vi "Get Brewer Palette Colors by Name (#Colors).vi"(11 "Brewer Palette Name (# Colors)":string) -> (0 "Found?":bool, 3 "Color Array":u32[](array[numeric]))   [LabVIEW 2021, in "Palette.lvlib"]
uses:
  Palette.lvlib
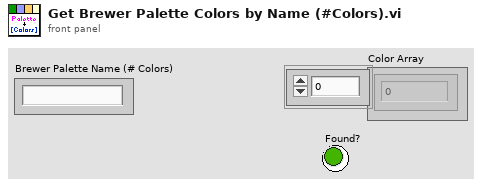
[diagram p1: front panel]
types:
  T1 = typedef "Palette.lvlib/Color Brewer Palette.ctl" = cluster{"Color Array":u32[], "Palette Name":string, "Number of Colors":i32, "Palette Category":string, "Color Blind Safe":bool, "Printer Friendly":bool, "Photocopy Safe":bool}
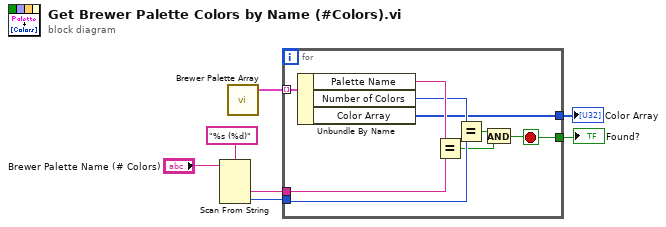
[diagram p0: block diagram]
diagram:
  n1 = Scan From String(format string="%s (%d)", input string="Brewer Palette Name (# Colors)") -> (output 1=w4:string, output 2=w3:i32)  [unwired: 4 in, 3 out]
  n2 = call "Brewer Palette Array.vi"() -> ("Color Brewer Palette Array"=w5:T1[])  [unwired: 9 in]
  n3 = for {
    tunnel: w5 -> [w16] mode=indexing
    tunnel: w4 -> [w14]
    tunnel: w3 -> [w12]
    tunnel: [w9] -> w2
    tunnel: [w8] -> w1
    stop <- w8 stop-if-true
    n4 = Unbundle By Name(w16) -> ("Palette Name"=w15:string, "Number of Colors"=w13:i32, "Color Array"=w9:u32[])
    n5 = Equal?(x=w15, y=w14) -> (x = y?=w10:bool)
    n6 = Equal?(x=w13, y=w12) -> (x = y?=w11:bool)
    n7 = And(x=w11, y=w10) -> (x .and. y?=w8:bool)
  }
  "Color Array" <- w2
  "Found?" <- w1
